vi "excavator1D.vi"(2 "Name":string="data_labView_Photon_Source_Mar1'18_rabi_temp") -> ()   [LabVIEW 2013]
panel:
  in  "Waveform Graph":dbl[][](graph)=[[3.7804722978762584e-05, 4.56032903457526e-05, 4.9491034587845206e-05, 5.4381299378292176e-05, 5.363908712752164e-05, 6.145102452137506e-05, 6.371047948050546e-05, 6.366143770719646e-05, 6.71379420964513e-05, 7.242772880999836e-05, 7.46241548768012e-05, 7.490970165235922e-05, 8.179236101568677e-05, 7.953111344249919e-05, 8.209020961658099e-05, 8.1527563452255e-05, 7.99810750322649e-05, 7.753344289085362e-05, 8.65301608428126e-05, 8.497790440742395e-05, 7.79496749601094e-05, 7.812280455254948e-05, 7.281845682882704e-05, 7.508642374887128e-05, 7.621411532454658e-05, 7.52975192881422e-05, 7.107558303687256e-05, 6.998146454861853e-05, 6.772905544494276e-05, 6.66369505779585e-05, 5.874692487850551e-05, 5.3532186939264654e-05, 5.093463823868659e-05, 4.841296686208807e-05, 4.9043344006349785e-05, 4.611730491888012e-05, 4.1388569115952137e-05, 3.442570505285403e-05, 2.6823670395970112e-05, 2.957886908916408e-05, 2.3737029550829902e-05, 2.220908254457754e-05, 1.3019855032325732e-05, 1.3343350360628394e-05, 4.247169613336158e-06, 2.3744121335764647e-08, -1.0549078695021253e-06, -3.183061267009188e-06, -1.226291942657554e-05, -9.262793469133607e-06, -2.1582135104836198e-05, -2.268091770929459e-05, -2.5415661639272e-05, -3.2467311029904515e-05, -3.601735443226062e-05, -3.788469166465802e-05, -3.908792677975726e-05, -4.383123541629175e-05, -4.9979953473666676e-05, -4.985502346244175e-05, -5.0357140025880653e-05, -5.49290862181806e-05, -5.9588615840766586e-05, -6.433004909922602e-05, -6.648815360676963e-05, -6.694961302855518e-05, -6.647637746937107e-05, -7.395179272862151e-05, -7.750596705591306e-05, -7.284923594852444e-05, -7.709854435233865e-05, -7.979991460160818e-05, -8.125903150357772e-05, -8.165308281604666e-05, -7.814034688635729e-05, -8.238861119025387e-05, -8.223569057008717e-05, -8.424065890721977e-05, -8.040250759222545e-05, -7.949092287162784e-05, -8.08051318017533e-05, -8.228885781136341e-05, -8.019716187845916e-05, -8.332198376592714e-05, -7.873120193835348e-05, -8.270555736089591e-05, -7.088447819114663e-05, -8.096270357782487e-05, -7.418351196974982e-05, -7.456550702045206e-05, -7.39644056011457e-05, -6.757125811418518e-05, -6.350509192998288e-05, -6.663423482677899e-05, -6.43139319436159e-05, -5.879550008103252e-05, -5.6706058785493945e-05, -5.206004061619751e-05, -5.653227344737388e-05, -4.865002483711578e-05, -4.523999359662411e-05, -4.207868914818391e-05, -3.5842048418999184e-05, -3.846434265142307e-05, -3.0097996841504934e-05, -3.483676391624613e-05, -2.5430529149161885e-05, -2.6761739263747593e-05, -1.889204713734216e-05, -1.7356212538288673e-05, -1.8881057940234317e-05, -1.2915116712974848e-05, -4.273522890230199e-06, -7.737443070254812e-06, -4.323300515807199e-06, 1.5055955771003982e-06, 3.47920774856903e-06, 1.0270843233683931e-06, 8.079278245531899e-06, 1.0162324201701282e-05, 7.607411760091051e-06, 1.202828207169659e-05, 9.592143214831598e-06, 1.5906048247416035e-05, 1.5011407299425641e-05, 1.6472288962177114e-05, 1.743462621561775e-05, 2.389577412031939e-05, 2.3391452486976043e-05, 2.2365841232385712e-05, 1.9737952925424923e-05, 2.1284297417878406e-05, 2.4709215722396052e-05, 2.834958468156401e-05, 2.7961878458881987e-05, 2.0035314946653684e-05, 2.2764344976167198e-05, 2.543647588026943e-05, 1.897152651508804e-05, 2.516713129807613e-05, 2.0830328139709316e-05, 2.0296283764764667e-05, 2.0299291463743443e-05, 1.770115864019317e-05, 1.4098381370786215e-05, 1.9532106762198974e-05, 1.629759162824484e-05, 1.4314760164779732e-05, 1.2334295661275984e-05, 1.4293294270828484e-05, 1.0201850045632458e-05, 1.5466010154341348e-05, 6.159797159455138e-06, 4.757488540008136e-06, 5.906744206640724e-06, 6.277824866174337e-06, 1.1711202432707072e-05, 4.3423017426214025e-06, -1.833961334796183e-06, -6.3195533641646745e-06, -1.7968321230910112e-06, -3.4872696517140862e-06, -5.913458323902889e-06, -1.2042905154885372e-05, -5.589133536432205e-06, -1.3502842080015407e-05, -1.0528526331654575e-05, -1.6305303461194853e-05, -1.8083632767229574e-05, -1.647801263970905e-05, -1.901145787996938e-05, -1.9542467725841565e-05, -2.026369384111603e-05, -2.8099093015043763e-05, -2.344849804103433e-05, -2.4168494746845674e-05, -2.8206478873471497e-05, -3.106418580500758e-05, -3.0139574391796483e-05, -2.8857503821200222e-05, -2.7708076686394634e-05, -3.101750826317584e-05, -3.4478443467378384e-05, -3.4880798011727165e-05, -2.9828828246536435e-05, -3.579832264222205e-05, -3.381249689482502e-05, -3.574256606952985e-05, -4.057531896251021e-05, -3.9560226468893234e-05, -3.6041811654285993e-05, -3.4048024645016994e-05, -3.8454230889328755e-05, -3.3567390346433974e-05, -3.8639310332655434e-05, -3.838176144199679e-05, -3.6268338590161875e-05, -3.3936465115402825e-05, -3.542535978340311e-05, -3.7119867556612e-05, -3.551014151526033e-05, -3.677779568533878e-05, -3.188626442351961e-05, -3.037659280380467e-05, -3.266771454946138e-05, -3.1589560421707574e-05, -3.1227849376591614e-05, -2.6031908419099636e-05, -2.9668714432773413e-05, -2.211146056652069e-05, -2.7014504667022272e-05, -2.6552392682788195e-05, -2.5561170332366597e-05, -2.252192280138843e-05, -2.3258693090610905e-05, -2.001221173486556e-05, -1.6096717672553496e-05, -1.739483332130477e-05, -1.613346944395744e-05, -1.6128531342474155e-05, -1.71508120274666e-05, -1.2784274645127878e-05, -1.412635606357071e-05, -7.808507518802795e-06, -1.2962803793925563e-05, -7.646931891258644e-06, -2.312037807428173e-06, -6.2482103260208516e-06, -2.1407375356829965e-06, -5.709832123557144e-06, -5.695087565982254e-06, -5.762534470932224e-06, -3.5473104631478194e-06, 2.396438148366536e-06, -3.952478436985984e-06, -1.399290283643499e-06, 3.1178746695559005e-07, 4.277902689864264e-06, 1.0232834597445653e-06, 2.7990138491418183e-06, 4.272691057849432e-06, 2.7727228015805765e-06, 6.332420724675098e-06, 3.0738521630269066e-06, 4.173143281605011e-06, 8.896997314877801e-06, 3.2173065778184783e-06, 4.903221679342093e-06, 2.4765658963587986e-06, 2.4964562186369323e-06, 5.308589635433243e-06], [0.00017391681467415765, 0.00018473039381206036, 0.00020287145889597014, 0.0002175243898818735, 0.00023411940128426068, 0.00024701488655409776, 0.00026087070000357926, 0.00026398643240099773, 0.00027892927755601704, 0.0002847738651325926, 0.00029634492966579273, 0.0002989494023495354, 0.00030426889861701056, 0.00030851650080876425, 0.0003139787440886721, 0.000318953265377786, 0.00031971913995221257, 0.0003193069569533691, 0.00032568766619078815, 0.00032368848769692704, 0.00032063430262496695, 0.0003158190520480275, 0.00031742610735818744, 0.00031333702645497397, 0.0003105861251242459, 0.00030570782109862193, 0.0002985850442200899, 0.0002998194977408275, 0.0002912796917371452, 0.00028416271379683167, 0.00028508249670267105, 0.0002697963936952874, 0.0002658635421539657, 0.00025832478422671556, 0.0002498573376215063, 0.00023784672521287575, 0.000231682657613419, 0.00022053570864954963, 0.00020942764604114927, 0.00020344242875580676, 0.000195772634469904, 0.00018300580268260092, 0.00017423860117560253, 0.000164755907462677, 0.00015197095854091458, 0.00014501303667202592, 0.00014120641935733147, 0.0001282307530345861, 0.00012014114508929197, 0.00011574366362765431, 0.00010694862794480287, 0.00010008825302065816, 8.674748096382245e-05, 7.556000309705269e-05, 7.126170930860098e-05, 5.928372866037534e-05, 5.098809742776211e-05, 4.656346663978184e-05, 3.882375312969089e-05, 3.32938279825612e-05, 2.0627406229323242e-05, 2.071941730719118e-05, 1.6460570805065796e-05, 3.816780008492055e-06, 1.0567200803279762e-06, -4.935352279744622e-06, -5.874693897567332e-06, -1.2172298056611908e-05, -1.711812001303769e-05, -2.2358380647347083e-05, -2.390704503341112e-05, -2.691168356250273e-05, -3.261253596065217e-05, -3.0785662147536634e-05, -3.3059578527172555e-05, -3.485246134005137e-05, -3.1165450764092384e-05, -3.3587690268177546e-05, -3.4823366149794304e-05, -3.4742382922559045e-05, -2.9589873065560817e-05, -3.0027784305275418e-05, -2.9458853532560176e-05, -2.0893913188047002e-05, -2.4361335363209946e-05, -1.9242123926233028e-05, -1.1825140063592707e-05, -7.513051059504502e-06, -4.845303767098123e-06, -1.163195818776329e-06, 7.352432305651747e-06, 1.1994057331321525e-05, 1.8771065924738654e-05, 2.833903045029728e-05, 3.099604737144545e-05, 4.01473780584638e-05, 4.195933615847026e-05, 5.437802610686049e-05, 5.8546356740407646e-05, 6.391025362972869e-05, 7.138510045479053e-05, 8.180125769285951e-05, 8.644157060189173e-05, 9.738813605508767e-05, 0.00010460031990078278, 0.00011323348371661268, 0.00011732023631338961, 0.00012463205530366395, 0.00013237405801191926, 0.00013813036639476195, 0.00014724774518981576, 0.00015041601727716625, 0.0001551779714645818, 0.00016365815463359468, 0.00016991980373859406, 0.0001763684776960872, 0.0001815760406316258, 0.00018400368935544975, 0.00018857185204979032, 0.00019394472838030197, 0.00019529677229002118, 0.00020404640963533893, 0.00020627101912396029, 0.0002073621581075713, 0.00020633763415389694, 0.00021396537704276852, 0.00021299372383509763, 0.00021839347391505726, 0.0002171076921513304, 0.00021904451568843797, 0.00021829028992215171, 0.00021518855646718293, 0.00021925228065811098, 0.0002235368374385871, 0.0002172884087485727, 0.00021644380831276067, 0.00022234271091292612, 0.0002120541212207172, 0.00021291110897436738, 0.0002107287546095904, 0.00020577571922331117, 0.00020993170983274467, 0.00020513200797722675, 0.00020377741020638496, 0.00019928643087041564, 0.00019648018496809527, 0.00018914501924882643, 0.000191090366570279, 0.0001867010178102646, 0.0001842312231019605, 0.00018345025819144212, 0.00017945854051504284, 0.00017298312377533875, 0.00016861916810739785, 0.00016687500828993507, 0.00016396244973293506, 0.0001624514588911552, 0.00015580646868329495, 0.00015233645535772666, 0.00014651954552391544, 0.00014505034050671384, 0.00013823383051203564, 0.00013821033280692063, 0.00013758755449089222, 0.00013350305744097568, 0.00012621652604138944, 0.00012321976100793108, 0.00011909386375918984, 0.00011799447383964434, 0.00011174804785696324, 0.00011508412717375904, 0.00011145683129143436, 0.00010473850306880195, 0.00010204172940575518, 0.00010262300384056289, 9.903707541525364e-05, 9.444705938221887e-05, 9.666708137956448e-05, 8.922501729102805e-05, 8.928492752602324e-05, 8.399064608966e-05, 8.933044409786817e-05, 8.426576823694631e-05, 9.230969772033859e-05, 8.861105015967041e-05, 8.569366036681458e-05, 7.88201668910915e-05, 8.36302697280189e-05, 8.103447908069938e-05, 8.498914394294843e-05, 8.063355926424265e-05, 8.200984848372173e-05, 8.0149377026828e-05, 8.335821075888816e-05, 8.135177995427512e-05, 8.608642201579642e-05, 8.225159035646357e-05, 8.845287629810628e-05, 9.39495785132749e-05, 8.757015530136414e-05, 9.25475233088946e-05, 8.976754361356143e-05, 9.241909901902545e-05, 9.812481403059792e-05, 9.999064786825329e-05, 9.743731970957015e-05, 0.00010389933595433831, 0.00010989933070959523, 0.00011049005661334377, 0.0001130799028032925, 0.00011372593326086644, 0.00011792248551500961, 0.000116685458124266, 0.00012187116226414219, 0.00012519343545136508, 0.00012863168558396865, 0.00013324623796506785, 0.00013223573478171602, 0.00014032236140337773, 0.00013834701167070307, 0.0001421500273863785, 0.00014415825717151165, 0.00014736659431946464, 0.00014747883687959984, 0.00015318959776777774, 0.0001569411215314176, 0.000158684157213429, 0.0001614074280951172, 0.0001631251725484617, 0.00016219185636145994, 0.00016632328697596677, 0.00016738546037231572, 0.00016581940508331172, 0.00016849460735102184, 0.00017314657088718377, 0.0001717873674351722, 0.00017174651293316856, 0.00017484972340753302, 0.00017812017176765949, 0.0001757998288667295, 0.00017518529057269916, 0.0001747602982504759, 0.00018325658311368898, 0.0001776367389538791, 0.00018164664288633503, 0.0001779405320121441, 0.00017577845210325904, 0.00017725309226079844, 0.0001753736796672456, 0.00017759059119271114, 0.0001750500923662912], [0.0001779782444736049, 0.00019027605863144716, 0.00020882095522038632, 0.0002242190578776763, 0.00024018544028640566, 0.00025454387164899574, 0.0002685377949488551, 0.00027155407406767774, 0.00028689553002245963, 0.0002938399737325246, 0.00030559627260439624, 0.0003081918372812457, 0.00031507071108900157, 0.00031860261969526854, 0.00032453267055012204, 0.0003292080331608174, 0.00032957138955786087, 0.0003285854037009708, 0.0003369865348115341, 0.0003346572594536102, 0.00032997349567228214, 0.00032533804915452257, 0.00032567140078229665, 0.0003222081053900415, 0.00031980045730798604, 0.0003148443874230811, 0.00030692795105031475, 0.0003078784445295442, 0.0002990503030761722, 0.00029187142904832147, 0.0002910725529982331, 0.0002750559744660764, 0.0002706986524147458, 0.00026282220131900727, 0.0002546250945107975, 0.00024227643407370472, 0.00023535052048441, 0.0002232064693460858, 0.00021113845746298458, 0.00020558144691254466, 0.00019720641718560687, 0.00018434849379090387, 0.00017472437369953127, 0.00016529535396585308, 0.00015203029530185366, 0.00014501303861593146, 0.00014121035974152778, 0.0001282702533826395, 0.00012076536728809707, 0.00011611371586855453, 0.00010910452591418594, 0.00010262593444574855, 9.039403359807937e-05, 8.22401383360897e-05, 7.984660940755488e-05, 7.035488857501813e-05, 6.424680614040379e-05, 6.394789772644966e-05, 6.328727799728053e-05, 5.994999871703912e-05, 5.441811683011159e-05, 5.870688857633192e-05, 6.182033265073104e-05, 6.444317672757958e-05, 6.6496550492229e-05, 6.713127726178362e-05, 6.673545376964496e-05, 7.494686442911402e-05, 7.937383046100926e-05, 7.620307318904829e-05, 8.072008636937326e-05, 8.421558693372765e-05, 8.755916686837687e-05, 8.726386954075808e-05, 8.484603434406665e-05, 8.94571255704016e-05, 8.794313006067154e-05, 9.06896992534079e-05, 8.761980402352262e-05, 8.675159935194745e-05, 8.605248348266728e-05, 8.75963695034385e-05, 8.543657779202428e-05, 8.590173797426377e-05, 8.24140571707071e-05, 8.491447786784627e-05, 7.186406046108671e-05, 8.131054855831105e-05, 7.434157932652136e-05, 7.457457919244267e-05, 7.432894158226649e-05, 6.862748964082006e-05, 6.622121727200777e-05, 7.241009527554291e-05, 7.139353468417814e-05, 7.119496326811269e-05, 7.054192366134768e-05, 7.528092422545392e-05, 8.138534160832483e-05, 8.032026790087438e-05, 8.45132509584333e-05, 9.198946592171897e-05, 9.357776211788628e-05, 0.00010470890458738621, 0.00010884445937767037, 0.00011847118617941097, 0.00012004478190007242, 0.00012747289867903828, 0.00013371537188963176, 0.00013921650848238305, 0.00014845333547087246, 0.00015096946212143214, 0.00015523680564143248, 0.0001638409582593407, 0.00016997479410169115, 0.0001763749039485975, 0.00018160937040256355, 0.00018400655585773068, 0.00018874484926073278, 0.00019421078883442492, 0.00019544488220618099, 0.00020440062831280346, 0.00020649392858360517, 0.00020797131289165466, 0.0002068829659912499, 0.00021459850623130526, 0.0002137060892544247, 0.00021969687633076652, 0.00021836416839932167, 0.00022018340243355, 0.00021918083278421802, 0.00021623860929769845, 0.0002206402227958424, 0.00022532735440612282, 0.0002190801662027763, 0.0002173691238468396, 0.00022350502566676882, 0.00021357426022790797, 0.00021375467045893438, 0.00021222627668854668, 0.00020682734150077683, 0.000210910554330407, 0.0002061339417240621, 0.00020454477242801041, 0.000199784498613744, 0.00019744864213173732, 0.0001898458579993779, 0.00019162578259341505, 0.0001871080033051727, 0.00018478485280660003, 0.0001837337066922135, 0.00018012374977743347, 0.00017309276187096848, 0.00016868626959666637, 0.00016697951377006877, 0.00016408258898333977, 0.00016287304491009104, 0.0001558669665707989, 0.00015234749438416826, 0.000146655766934878, 0.00014506146933900883, 0.0001382778107566574, 0.00013833678138495308, 0.00013811360076166937, 0.00013362000134626748, 0.00012693674877747017, 0.0001236687485566503, 0.00012020487222261053, 0.00011937216438833021, 0.00011295641239166795, 0.00011664386764021414, 0.00011315711770075631, 0.00010668069794100486, 0.00010583984867896138, 0.00010526781548811857, 0.00010194340805140343, 9.856902391922105e-05, 0.00010153574869065267, 9.417801046477299e-05, 9.38325839467176e-05, 8.844301071434444e-05, 9.45622232267121e-05, 9.104659664422365e-05, 9.868004034836626e-05, 9.349693687475005e-05, 9.287046533241661e-05, 8.576656490149333e-05, 9.094807883631134e-05, 9.062529066871866e-05, 9.374521911236503e-05, 8.832204179559685e-05, 8.87968649815447e-05, 8.889685321246434e-05, 8.986301238881928e-05, 9.006169221545891e-05, 9.425514132858828e-05, 8.989280560900363e-05, 9.473961679222185e-05, 0.00010040657059478507, 9.511265250704267e-05, 9.912625394437239e-05, 9.70093714126897e-05, 9.776514574415078e-05, 0.00010271911467155265, 0.00010519177360895727, 0.00010243013033195701, 0.00010849078573058429, 0.00011294035216147226, 0.00011440404375070564, 0.00011522144377843422, 0.00011689042457985862, 0.00012087490288400912, 0.0001194523736324653, 0.00012393472958894362, 0.000127335631637018, 0.0001301791041400042, 0.00013421499264863588, 0.00013337492185390892, 0.00014124678384345345, 0.00013928397309625692, 0.00014318093671697237, 0.00014472401593698867, 0.00014804211244423814, 0.0001476854092895802, 0.00015373707147742, 0.00015712730887687453, 0.00015870099958525537, 0.00016152831942590942, 0.00016313921869422473, 0.00016229233023422782, 0.00016642076136370125, 0.00016748462361536583, 0.00016585734386425396, 0.00016851164832786477, 0.00017319167732828675, 0.00017179306628500686, 0.00017174679594137292, 0.000174902047521219, 0.00017812311107652344, 0.00017582210983860667, 0.00017523738734047842, 0.00017478229268529948, 0.0001833659586911886, 0.00017766333215745093, 0.00018169457338270876, 0.00017816281737216054, 0.00017580789312608637, 0.00017732089639648196, 0.00017539116539514948, 0.00017760813712729557, 0.00017513056832364963]]
  in  "Tab Control":enum32{"Page 1", "Page 2"}(tab)
  in  "Limits":bool=TRUE
  in  "x Max":dbl=52.0 format="%#_13g"
  in  "x Min":dbl=2.0 format="%#_13g"
  in  "All data or only selected?":bool
  in  "Ring":u16(ring)=1 items=["Windows", "Mac"]
  out "xPoints":i32=251
  out "Different waveforms":i32=3
  # "All Data"
  # "Data on graph"
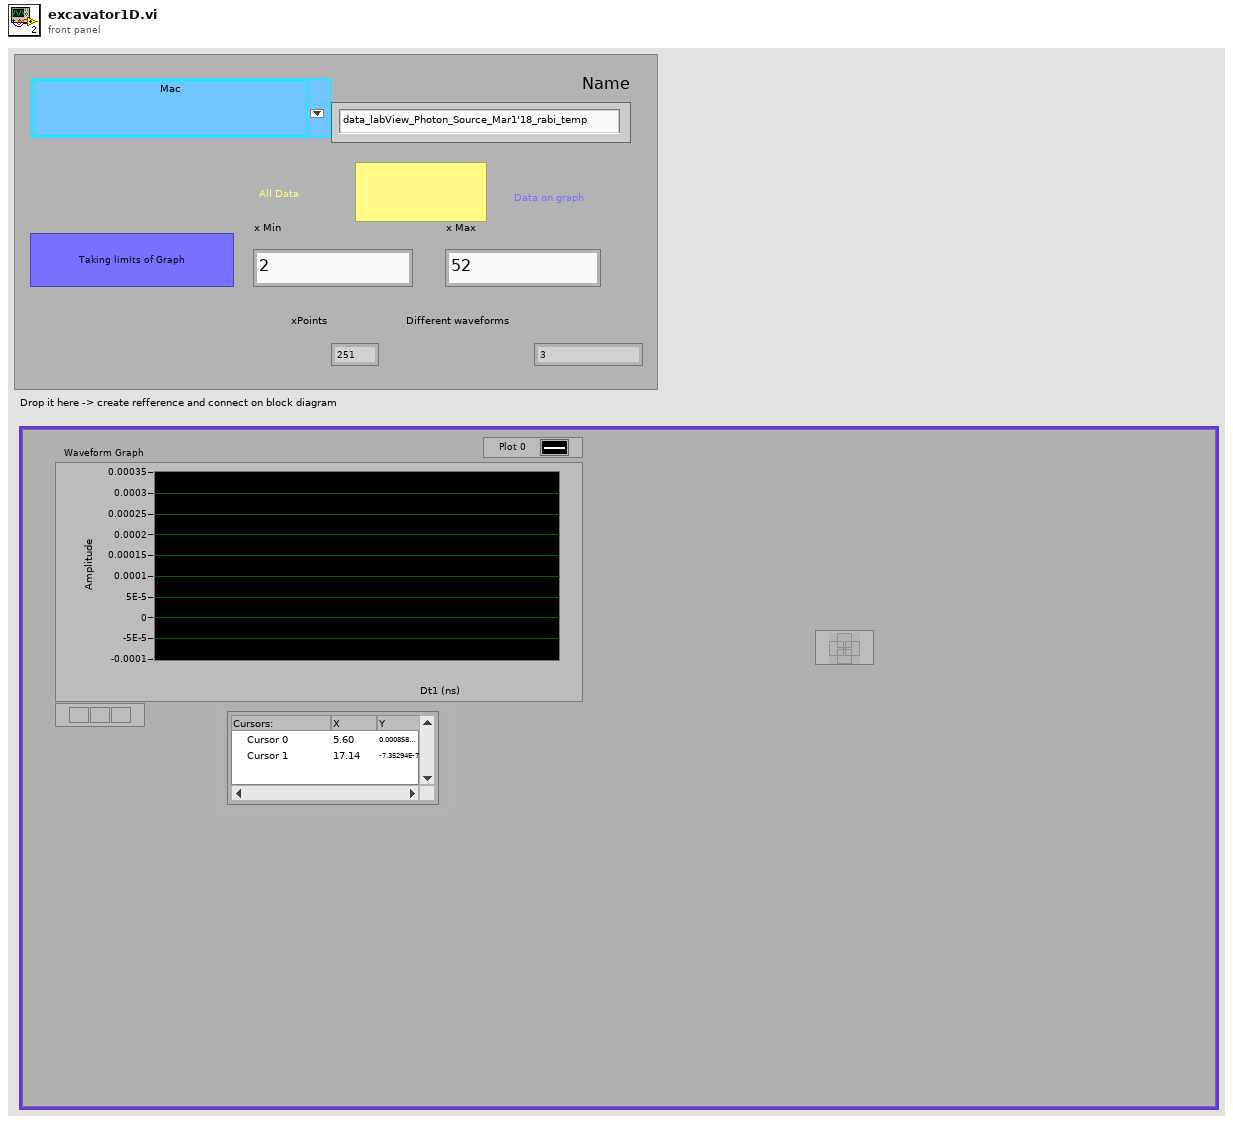
[diagram p1: front panel]
types:
  T1 = enum16{"open", "replace", "create", "open or create", "replace or create", "replace or create with confirmation"}
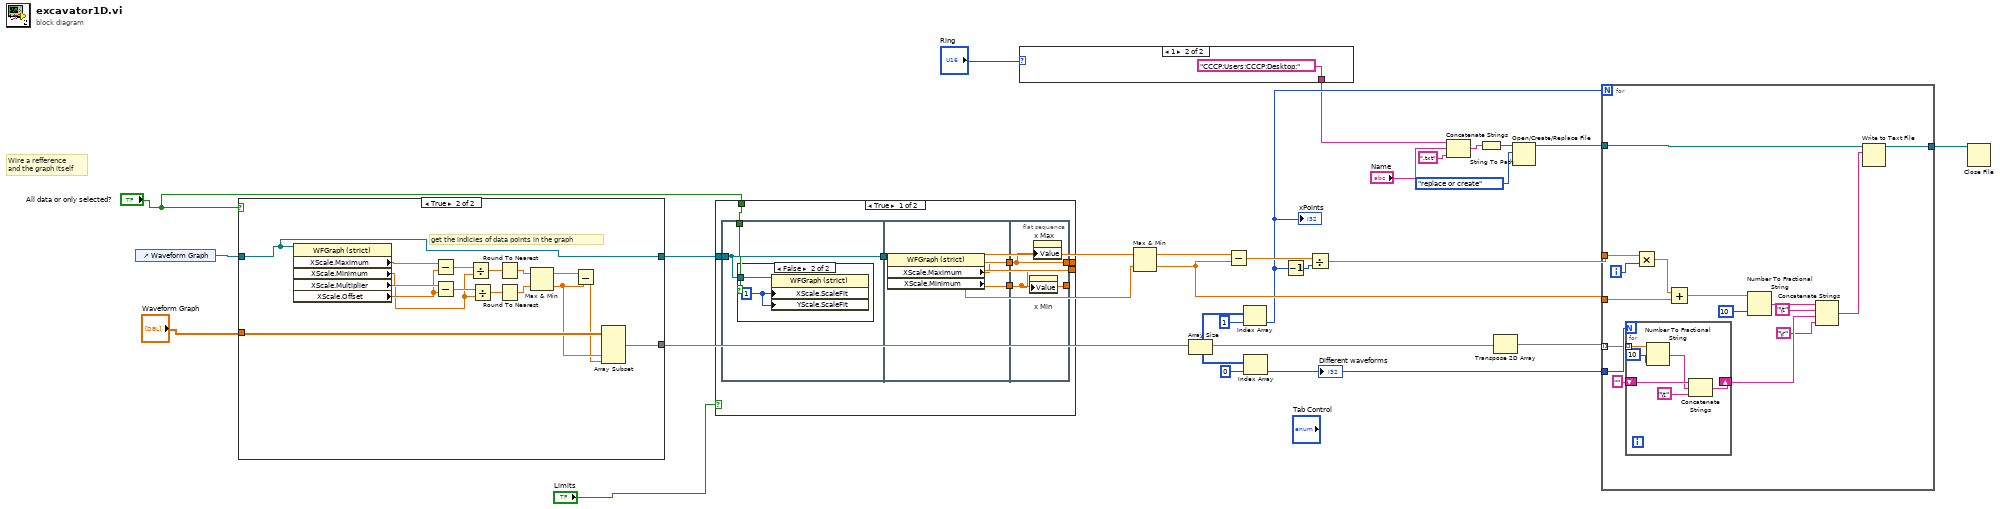
[diagram p0: block diagram]
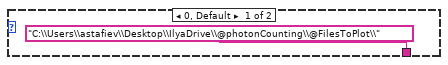
[diagram p2: hidden frame]
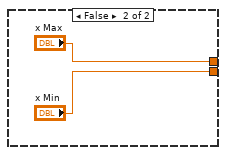
[diagram p5: hidden frame]
diagram:
  # "Wire a refference\nand the graph itself"
  n1 = control-ref of="Waveform Graph"() -> (w3:refnum<vi>)
  n2 = case shown="True" "All data or only selected?" {
    tunnel: "Waveform Graph" -> [w30 w35]
    tunnel: w3 -> [w29 w33]
    tunnel: [w30 w34] -> w14
    tunnel: [w29 w33] -> w16
    frame False {
    }
    frame True {
      # "get the indicies of data points in the graph"
      n3 = property class="WFGraph (strict)"(reference=w33) -> ("XScale.Maximum"=w43:dbl, "XScale.Minimum"=w46:dbl, "XScale.Multiplier"=w39:dbl, "XScale.Offset"=w40:dbl)  [unwired: 1 in, 2 out]
      n4 = Subtract(x=w43, y=w40) -> (x-y=w44:dbl)
      n5 = Subtract(x=w46, y=w40) -> (x-y=w45:dbl)
      n6 = Divide(x=w44, y=w39) -> (x/y=w42:dbl)
      n7 = Divide(x=w45, y=w39) -> (x/y=w41:dbl)
      n8 = Round To Nearest(number=w42) -> (nearest integer value=w38:dbl)
      n9 = Round To Nearest(number=w41) -> (nearest integer value=w37:dbl)
      n10 = Max & Min(x=w38, y=w37) -> (max(x,y)=w36:dbl, min(x,y)=w32:dbl)
      n11 = Subtract(x=w36, y=w32) -> (x-y=w31:dbl)
      n12 = Array Subset(array=w35, index (col)=w32, length (col)=w31) -> (w34:dbl[][])  [unwired: 2 in]
    }
  }
  n13 = case shown="True" "Limits" {
    tunnel: [w52 "x Max"] -> w11
    tunnel: [w51 "x Min"] -> w10
    tunnel: w16 -> [w53 _]
    tunnel: "All data or only selected?" -> [w49 _]
    frame True {
      n14 = flat-sequence {
        tunnel: w53 -> [w54]
        tunnel: [w54] -> w50
        tunnel: w49 -> [w55]
        tunnel: w50 -> [w60]
        tunnel: [w59] -> w48
        tunnel: [w58] -> w47
        tunnel: [w61] -> w51
        tunnel: [w62] -> w52
        tunnel: w48 -> [w62]
        tunnel: w47 -> [w61]
        frame #0 {
          n15 = case shown="False" w55 {
            tunnel: w54 -> [_ w56]
            frame True {
            }
            frame False {
              w57 = u8 1 ("X Scale.Scale Fit")
              n16 = property class="WFGraph (strict)"(reference=w56, "XScale.ScaleFit"=w57, "YScale.ScaleFit"=w57) -> ()  [unwired: 1 in, 2 out]
            }
          }
        }
        frame #1 {
          n17 = property class="WFGraph (strict)"(reference=w60) -> ("XScale.Maximum"=w59:dbl, "XScale.Minimum"=w58:dbl)  [unwired: 1 in, 2 out]
        }
        frame #2 {
          n18 = property on="x Min" class="DigNum (strict)"("Value"=w61) -> ()  [unwired: 2 in, 2 out]
          n19 = property on="x Max" class="DigNum (strict)"("Value"=w62) -> ()  [unwired: 2 in, 2 out]
        }
      }
    }
    frame False {
    }
  }
  n20 = case shown="1" "Ring" {
    tunnel: ["C:\\Users\\astafiev\\Desktop\\IlyaDrive\\@photonCounting\\@FilesToPlot\\" ("Directory") "CCCP:Users:CCCP:Desktop:" ("Directory")] -> w5
    frame 0, Default {
    }
    frame 1 {
    }
  }
  n21 = Max & Min(x=w11, y=w10) -> (max(x,y)=w9:dbl, min(x,y)=w8:dbl)
  n22 = Array Size(array=w14) -> (size(s)=w17:i32[])
  n23 = Subtract(x=w9, y=w8) -> (x-y=w20:dbl)
  n24 = Index Array(array=w17, index=1) -> (element=w6:i32)
  "xPoints" <- w6
  n25 = Index Array(array=w17, index=0) -> (element=w12:i32)
  "Different waveforms" <- w12
  n26 = Decrement(x=w6) -> (x-1=w7:i32)
  n27 = Divide(x=w20, y=w7) -> (x/y=w22:dbl)
  n28 = Concatenate Strings(w5, "Name", ".txt" ("FileName 2")) -> (w28:string)
  n29 = String To Path(string=w28) -> (path=w27:path)
  n30 = Transpose 2D Array(2D array=w14) -> (transposed array=w13:dbl[][])
  n31 = Open/Create/Replace File(file path (use dialog)=w27, operation (0:open)=T1."replace or create") -> (refnum out=w24:refnum<file>)  [unwired: 4 in, 2 out]
  n32 = for {
    N: w6 -> [_]
    tunnel: w13 -> [w72] mode=indexing
    tunnel: w24 -> [w82]
    tunnel: w22 -> [w81]
    tunnel: w8 -> [w78]
    tunnel: [w76] -> w21
    tunnel: w12 -> [w73]
    i -> [w80]
    n33 = for {
      N: w73 -> [_]
      tunnel: w72 -> [w88] mode=indexing
      shift-right: [w84] -> w68
      shift-left: "" ("string") -> [w87]
      n34 = Number To Fractional String(number=w88, precision (6)=i16 10 ("width (-)")) -> (F-format string=w86:string)  [unwired: 2 in]
      n35 = Concatenate Strings(w87, w86, "\t") -> (w84:string)
    }
    n36 = Multiply(x=w81, y=w80) -> (x*y=w79:dbl)
    n37 = Add(x=w79, y=w78) -> (x+y=w77:dbl)
    n38 = Number To Fractional String(number=w77, precision (6)=i16 10 ("width (-)")) -> (F-format string=w75:string)  [unwired: 2 in]
    n39 = Concatenate Strings(w75, "\t", w68, "\r") -> (w74:string)
    n40 = Write to Text File(file (use dialog)=w82, text=w74) -> (refnum out=w76:refnum<file>)  [unwired: 2 in, 2 out]
  }
  n41 = Close File(refnum=w21) -> ()  [unwired: 1 in, 2 out]
